vi "Prime BSI Set File Name.vi"(7 "Requested File Path":path) -> (4 "File Path":string, 15 "File Name":string)   [LabVIEW 2025]
uses:
  kernel32.dll
  shell32.dll
panel:
  out "ReName Success?":bool
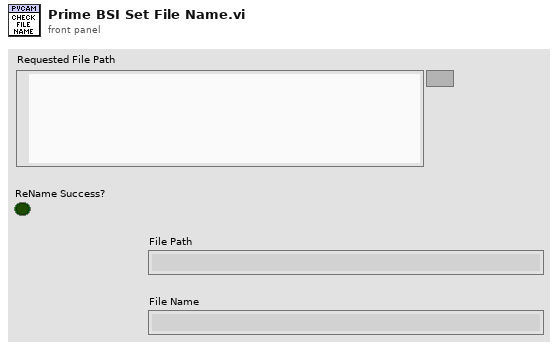
[diagram p1: front panel]
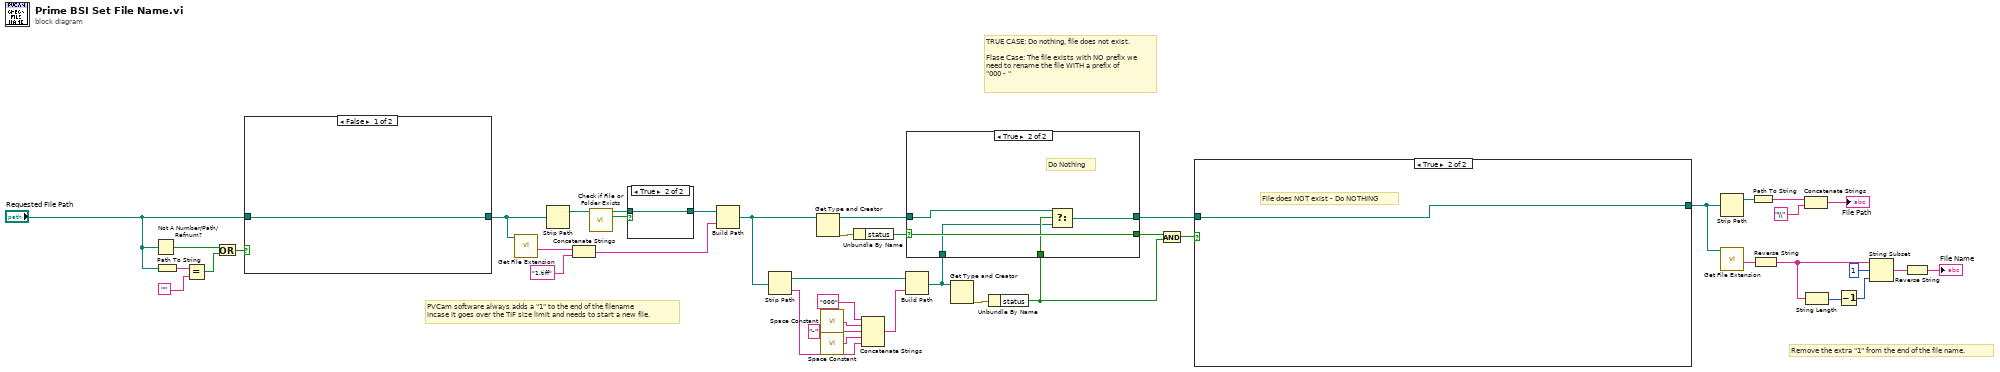
[diagram p0: block diagram]
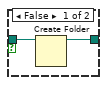
[diagram p2: hidden frame]
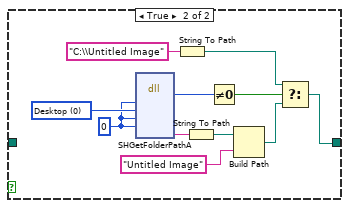
[diagram p3: hidden frame]
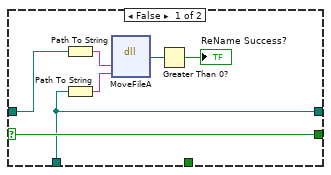
[diagram p4: hidden frame]
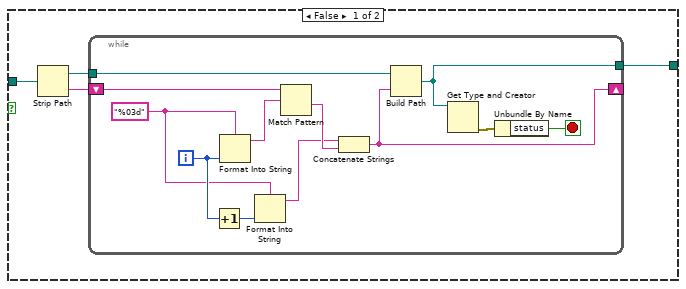
[diagram p5: hidden frame]
diagram:
  # "Remove the extra \"1\" from the end of the file name."
  # "PVCam software always adds a \"1\" to the end of the filename\nincase it goes over the TIF size limit and needs to start a new file."
  # "TRUE CASE: Do nothing, file does not exist.\n\nFlase Case: The file exists with NO prefix we\nneed to rename the file WITH a prefix of\n\"000 - \""
  n1 = Not A Number/Path/Refnum?(number/path/refnum="Requested File Path") -> (NaN/Path/Refnum?=w24:bool)
  n2 = Path To String(path="Requested File Path") -> (string=w26:string)
  n3 = Equal?(x=w26, y="") -> (x = y?=w23:bool)
  n4 = Or(x=w24, y=w23) -> (x .or. y?=w22:bool)
  n5 = case shown="False" w22 {
    tunnel: "Requested File Path" -> [w44 _]
    tunnel: [w44 w45] -> w12
    frame False {
    }
    frame True {
      w55 = 0 items=["Desktop"=0, "Personal Documents"=5, "AppData"=26, "Local AppData"=28, "Common AppData"=35, "Program Files"=38, "Program Files Common"=43, "Common Documents"=46] ("Requested Path")
      w54 = 0 ("HWND")
      n6 = dll-call lib="shell32.dll" fn="SHGetFolderPathA"("HWND"=w54, "nFolder"=w55, "hToken"=w54, "dwFlags"=w54) -> ("Succeeded"=w50:i32, "pszPath"=w53:string)  [unwired: 8 in, 2 out]
      n7 = String To Path(string="C:\\Untitled Image" ("regular expression")) -> (path=w47:path)
      n8 = String To Path(string=w53) -> (path=w52:path)
      n9 = Not Equal To 0?(x=w50) -> (x != 0?=w48:bool)
      n10 = Build Path(base path=w52, name or relative path="Untitled Image" ("regular expression")) -> (appended path=w46:path)
      n11 = Select(t=w47, s=w48, f=w46) -> (s? t:f=w45:path)
    }
  }
  n12 = call <vilib>:"Get File Extension.vi"("file"=w12) -> ("filename without extension"=w11:string)  [unwired: 6 in, 4 out]
  n13 = Strip Path(path=w12) -> (stripped path=w18:path)  [unwired: 1 out]
  n14 = Concatenate Strings(w11, "1.tiff" ("string")) -> (w9:string)
  n15 = call <vilib>:"Check if File or Folder Exists.vi"("path"=w18) -> ("file or folder exists?"=w20:bool, "dup path"=w19:path)  [unwired: 8 in, 1 out]
  n16 = case shown="True" w20 {
    tunnel: [w56 w58] -> w17
    tunnel: w19 -> [w57 w58]
    frame False {
      n17 = Create Folder(path (use dialog)=w57) -> (created path=w56:path)  [unwired: 2 in, 2 out]
    }
    frame True {
    }
  }
  n18 = Build Path(base path=w17, name or relative path=w9) -> (appended path=w27:path)
  n19 = Strip Path(path=w27) -> (stripped path=w40:path, name=w36:string)
  n20 = Get Type and Creator(7:w27) -> (0:w43:errorcluster, 3:w31:path)  [unwired: 1 in, 2 out]
  n21 = call <vilib>:"Space Constant.vi"() -> ("String"=w42:string)
  n22 = call <vilib>:"Space Constant.vi"() -> ("String"=w38:string)
  n23 = Unbundle By Name(w43) -> ("status"=w33:bool)
  n24 = Concatenate Strings("000", w42, "-", w38, w36) -> (w39:string)
  n25 = Build Path(base path=w40, name or relative path=w39) -> (appended path=w29:path)
  n26 = Get Type and Creator(7:w29) -> (0:w35:errorcluster)  [unwired: 1 in, 3 out]
  n27 = Unbundle By Name(w35) -> ("status"=w28:bool)
  n28 = case shown="True" w33 {
    selector: w33 -> [w65 w70]
    tunnel: [w65 w70] -> w32
    tunnel: w31 -> [w60 w68]
    tunnel: [w59 w67] -> w30
    tunnel: w29 -> [w59 w66]
    tunnel: w28 -> [_ w69]
    frame False {
      n29 = Path To String(path=w60) -> (string=w62:string)
      n30 = Path To String(path=w59) -> (string=w61:string)
      n31 = dll-call lib="kernel32.dll" fn="MoveFileA"(w62, w61) -> ("return type"=w63:i32)  [unwired: 5 in, 2 out]
      n32 = Greater Than 0?(x=w63) -> (x > 0?=→"ReName Success?":bool)
    }
    frame True {
      # "Do Nothing"
      n33 = Select(t=w68, s=w69, f=w66) -> (s? t:f=w67:path)
    }
  }
  n34 = And(x=w32, y=w28) -> (x .and. y?=w34:bool)
  n35 = case shown="True" w34 {
    tunnel: w30 -> [w74 w87]
    tunnel: [w71 w87] -> w2
    frame False {
      n36 = Strip Path(path=w74) -> (stripped path=w73:path, name=w72:string)
      n37 = while {
        tunnel: w73 -> [w85]
        tunnel: [w82] -> w71
        shift-right: [w75] -> _
        shift-left: w72 -> [w86]
        i -> [w79]
        stop <- w80 stop-if-true
        w77 = "%03d" ("format string")
        n38 = Increment(x=w79) -> (x+1=w78:i32)
        n39 = Format Into String(format string=w77, w79) -> (resulting string=w84:string)  [unwired: 2 in, 1 out]
        n40 = Format Into String(format string=w77, w78) -> (resulting string=w76:string)  [unwired: 2 in, 1 out]
        n41 = Match Pattern(string=w86, regular expression=w84) -> (after substring=w83:string)  [unwired: 1 in, 3 out]
        n42 = Concatenate Strings(w76, w83) -> (w75:string)
        n43 = Build Path(base path=w85, name or relative path=w75) -> (appended path=w82:path)
        n44 = Get Type and Creator(7:w82) -> (0:w81:errorcluster)  [unwired: 1 in, 3 out]
        n45 = Unbundle By Name(w81) -> ("status"=w80:bool)
      }
    }
    frame True {
      # "File does NOT exist - Do NOTHING"
    }
  }
  n46 = Strip Path(path=w2) -> (stripped path=w16:path)  [unwired: 1 out]
  n47 = call <vilib>:"Get File Extension.vi"("file"=w2) -> ("filename without extension"=w1:string)  [unwired: 6 in, 4 out]
  n48 = Path To String(path=w16) -> (string=w15:string)
  n49 = Reverse String(1:w1) -> (0:w3:string)
  n50 = Concatenate Strings(w15, "\\") -> (→"File Path":string)
  n51 = String Length(string=w3) -> (length=w7:i32)
  n52 = Decrement(x=w7) -> (x-1=w6:i32)
  n53 = String Subset(string=w3, offset (0)=1, length (rest)=w6) -> (substring=w5:string)
  n54 = Reverse String(1:w5) -> (0:→"File Name":string)
